vi "Display Data.vi"() -> ()   [LabVIEW 2011]
uses:
  <vilib>/Waveform/DWDTOps.llb/DWDT Binary U8 to Digital.vi
panel:
  out "Digital Waveform Graph":digitalwaveform[](graph)
  in  "Data":u64[](array[numeric])=[2233383036325, 4398046595914, 5566277700426, 4398046680724, 5566277785236, 4398046850344, 5566277954856, 4398047189584, 5566278294096, 4398047868064, 5566278972576, 4398049225024, 5566280329536, 4398051938944, 5566283043456, 4398057366784, 5566288471296, 4398068222464, 5566299326976, 4398089933824, 5566321038336, 4398133356544, 5566364461056, 4398220201984, 5566451306496, 4398393892864, 5566624997376, 4398741274624, 5566972379136, 4399436038144, 5567667142656, 4400825565184, 3370033414144, 1102290681856, 1133871408549, 1133871408549, 1133871408549, 1133871408549, 1133871408549, 1133871408549, 1133871408549, 1133871408549, 1133871408549, 1133871408549, 1133871408549, 1133871408549, 1133871408549, 1133871408549, 1133871408549, 1133871408549, 1133871408549, 1133871408549, 1133871408549, 1133871408549, 1133871408549, 1133871408549, 1133871408549, 1133871408549, 1133871408549, 1133871408549, 1133871408549, 1133871408549, 1133871408549, 1133871408549, 1133871408549, 1133871408549, 1133871408549, 1133871408549, 1133871408549, 1133871408549, 1133871408549, 1133871408549, 1133871408549, 1133871408549, 1133871408549, 1133871408549, 1133871408549, 1133871408549, 1133871408549, 1133871408549, 1133871408549, 1133871408549, 1133871408549, 1133871408549, 1133871408549, 1133871408549, 1133871408549, 1133871408549, 1133871408549, 1133871408549, 1133871408549, 1133871408549, 1133871408549, 1133871408549, 1133871408549, 1133871408549, 1133871408549, 1133871408549, 1133871408549, 1133871408549]
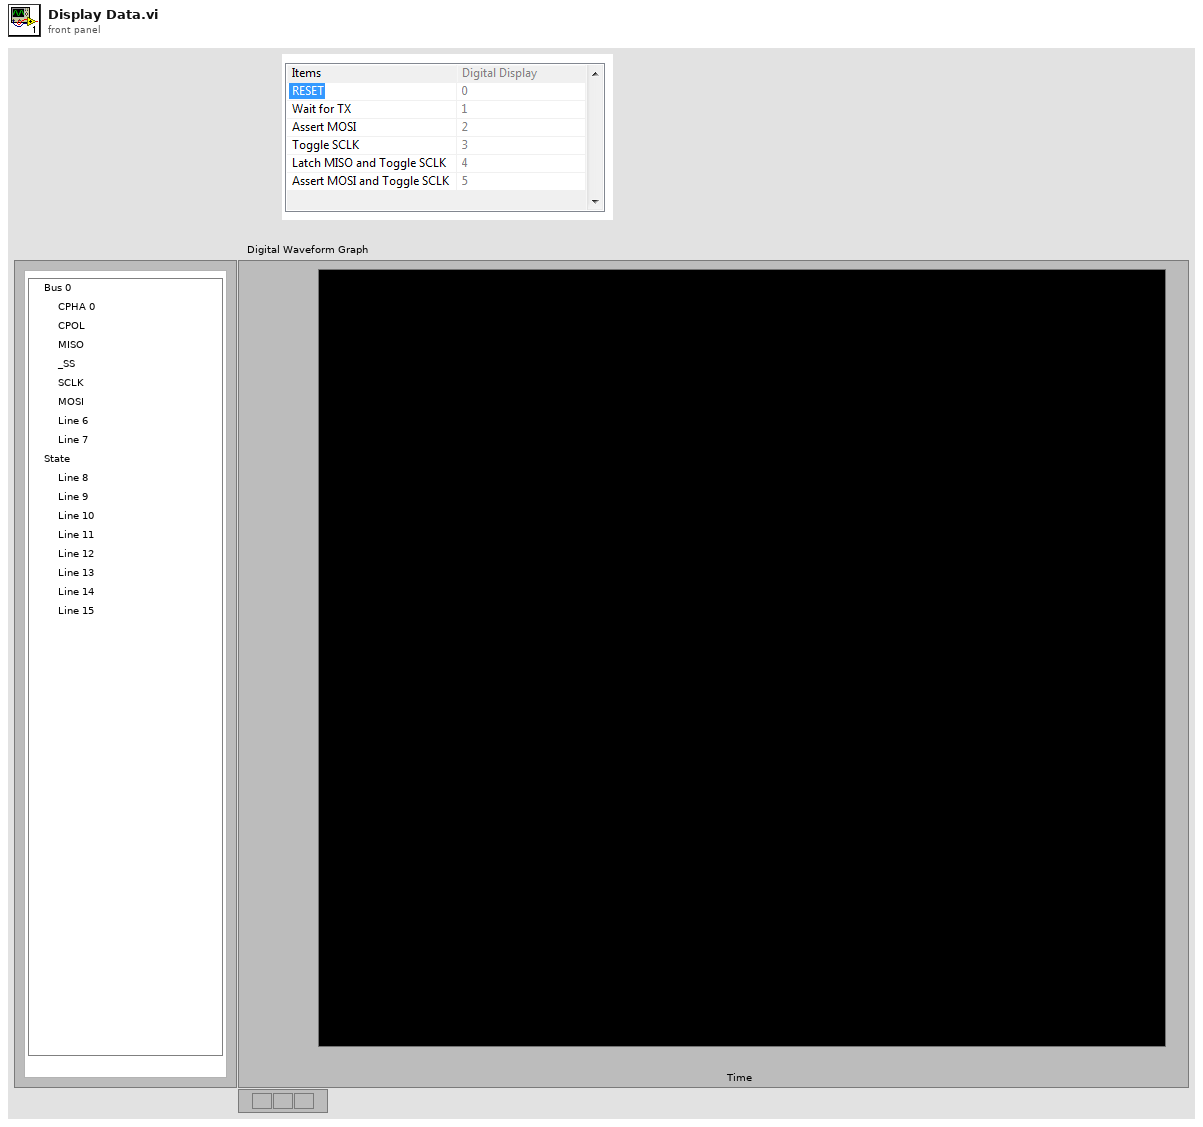
[diagram p1: front panel]
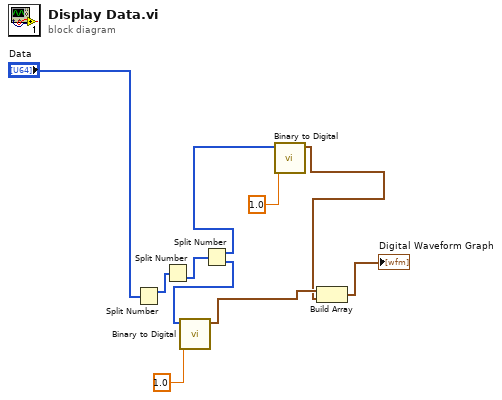
[diagram p0: block diagram]
diagram:
  n1 = Split Number(x="Data") -> (hi(x)=w8:u32[])  [unwired: 1 out]
  n2 = Split Number(x=w8) -> (lo(x)=w3:u16[])  [unwired: 1 out]
  n3 = Split Number(x=w3) -> (hi(x)=w6:u8[], lo(x)=w7:u8[])
  n4 = call-poly <vilib>:"Binary to Digital.vi"("sample rate"=1.0, "binary array"=w7) -> ("digital waveform"=w2:digitalwaveform)  [unwired: 8 in, 1 out]
  n5 = call-poly <vilib>:"Binary to Digital.vi"("sample rate"=1.0, "binary array"=w6) -> ("digital waveform"=w1:digitalwaveform)  [unwired: 8 in, 1 out]
  n6 = Build Array(w2, w1) -> (→"Digital Waveform Graph":digitalwaveform[])
